vi "GT Pvt Table Move Percent.vi"(0 "cardNum":i16, 1 "tableId":i16, 2 "distance":i32, 3 "vm":dbl, 4 "acc":dbl, 5 "pa1":dbl, 6 "pa2":dbl, 7 "error in (no error)":errorcluster caption="错误输入（无错误）", 8 "dec":dbl, 9 "pd1":dbl, 10 "pd2":dbl, 11 "pVel":dbl, 12 "pAcc":dbl, 13 "pDec":dbl, 14 "pTime":dbl) -> (15 "pDec out":dbl, 17 "pVel out":dbl, 20 "pAcc out":dbl, 21 "pTime out":dbl, 22 "function return":i16, 27 "error out":errorcluster caption="错误输出")   [LabVIEW 2014, in "gts.lvlib"]
doc: "GT_API GT_PvtTableMovePercent(short cardNum,short tableId,long distance,double vm,double acc,double pa1,double pa2,double dec,double pd1,double pd2,double *pVel,double *pAcc,double *pDec,double *pTime);"
uses:
  gts.lvlib
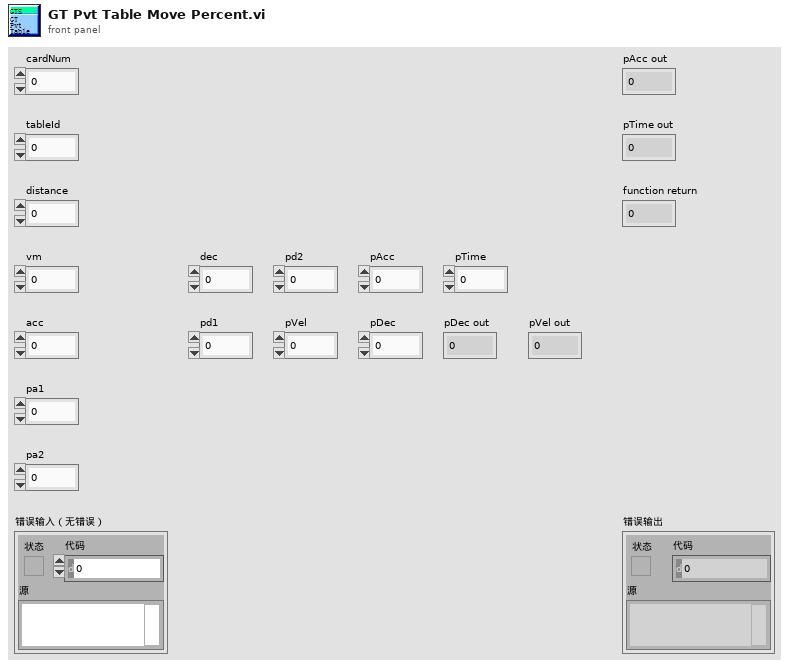
[diagram p1: front panel]
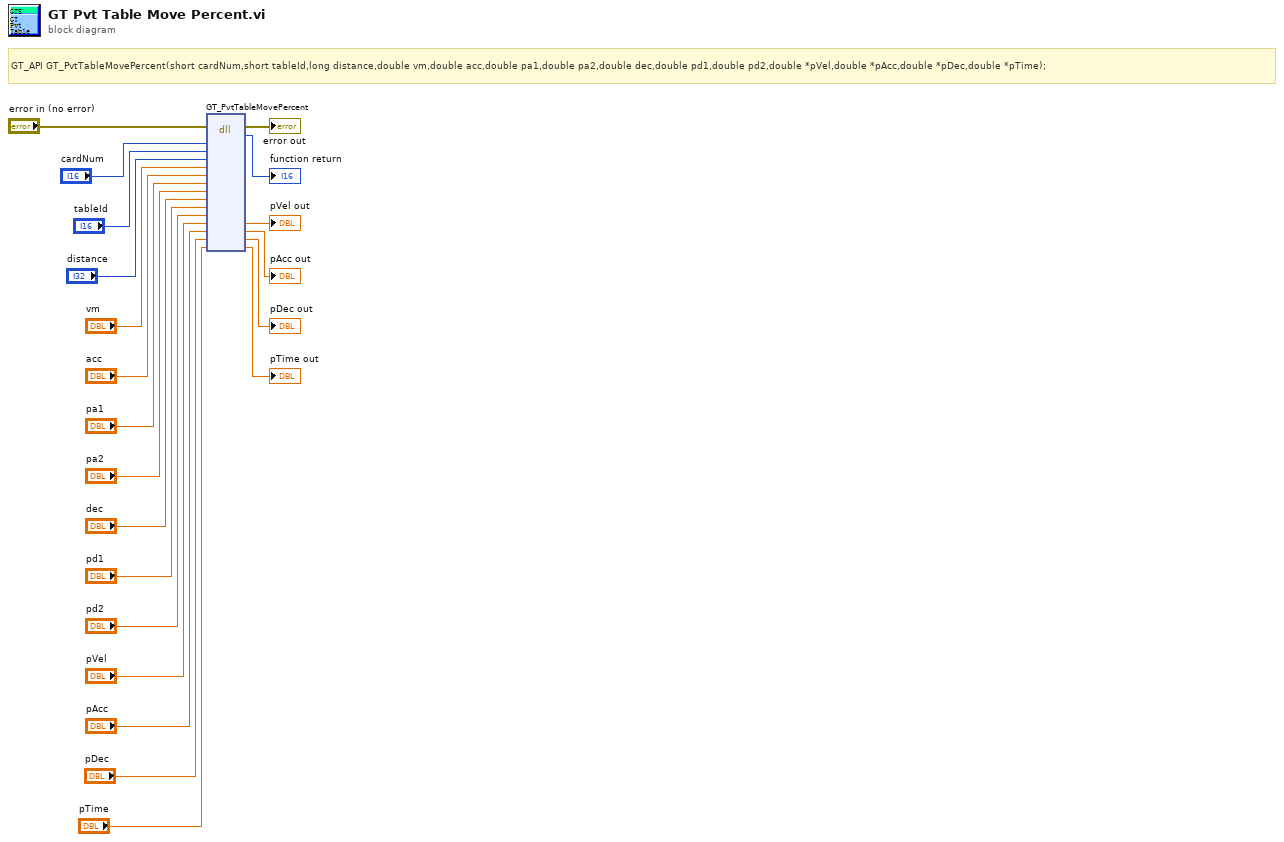
[diagram p0: block diagram]
diagram:
  # "GT_API GT_PvtTableMovePercent(short cardNum,short tableId,long distance,double vm,double acc,double pa1,double pa2,double dec,double pd1,double pd2,double *pVel,double *pAcc,double *pDec,double *pTime);"
  n1 = dll-call lib="PTH2habs D固高科技资料GTS控制卡GTS卡18年上半年资料dllVC32bit\nmulti_cardgts.*" fn="GT_PvtTableMovePercent"(error in="error in (no error)", "cardNum"="cardNum", "tableId"="tableId", "distance"="distance", "vm"="vm", "acc"="acc", "pa1"="pa1", "pa2"="pa2", "dec"="dec", "pd1"="pd1", "pd2"="pd2", "pVel"="pVel", "pAcc"="pAcc", "pDec"="pDec", "pTime"="pTime") -> (error out=→"error out":errorcluster, →"function return":i16, "pVel"=→"pVel out":dbl, "pAcc"=→"pAcc out":dbl, "pDec"=→"pDec out":dbl, "pTime"=→"pTime out":dbl)  [unwired: 12 in, 1 out]
